vi "MeasureLeakageThreshold.vi"(5 "Junction Name":string, 6 "UiDefinition":T1, 7 ".NET Refnum":refnum<k24>, 8 "new file path (Not A Path if cancelled)":path, 9 "appended path":path, 11 ".NET Refnum in":refnum<k24>) -> (0 "error out":errorcluster)   [LabVIEW 2020]
uses:
  UIReferences.ctl
  C:/Users/User/Desktop/Automation/CurrentVersion/LabviewDXFViewer/bin/Release/LabviewDXFViewer.exe
  LabviewDXFViewer/bin/Release/LabviewDXFViewer.exe
  <vilib>/Utility/file.llb/Write Delimited Spreadsheet (string).vi
  <vilib>/Utility/file.llb/Write Delimited Spreadsheet (DBL).vi
panel:
  in  "CurrentPositionIndex":i32
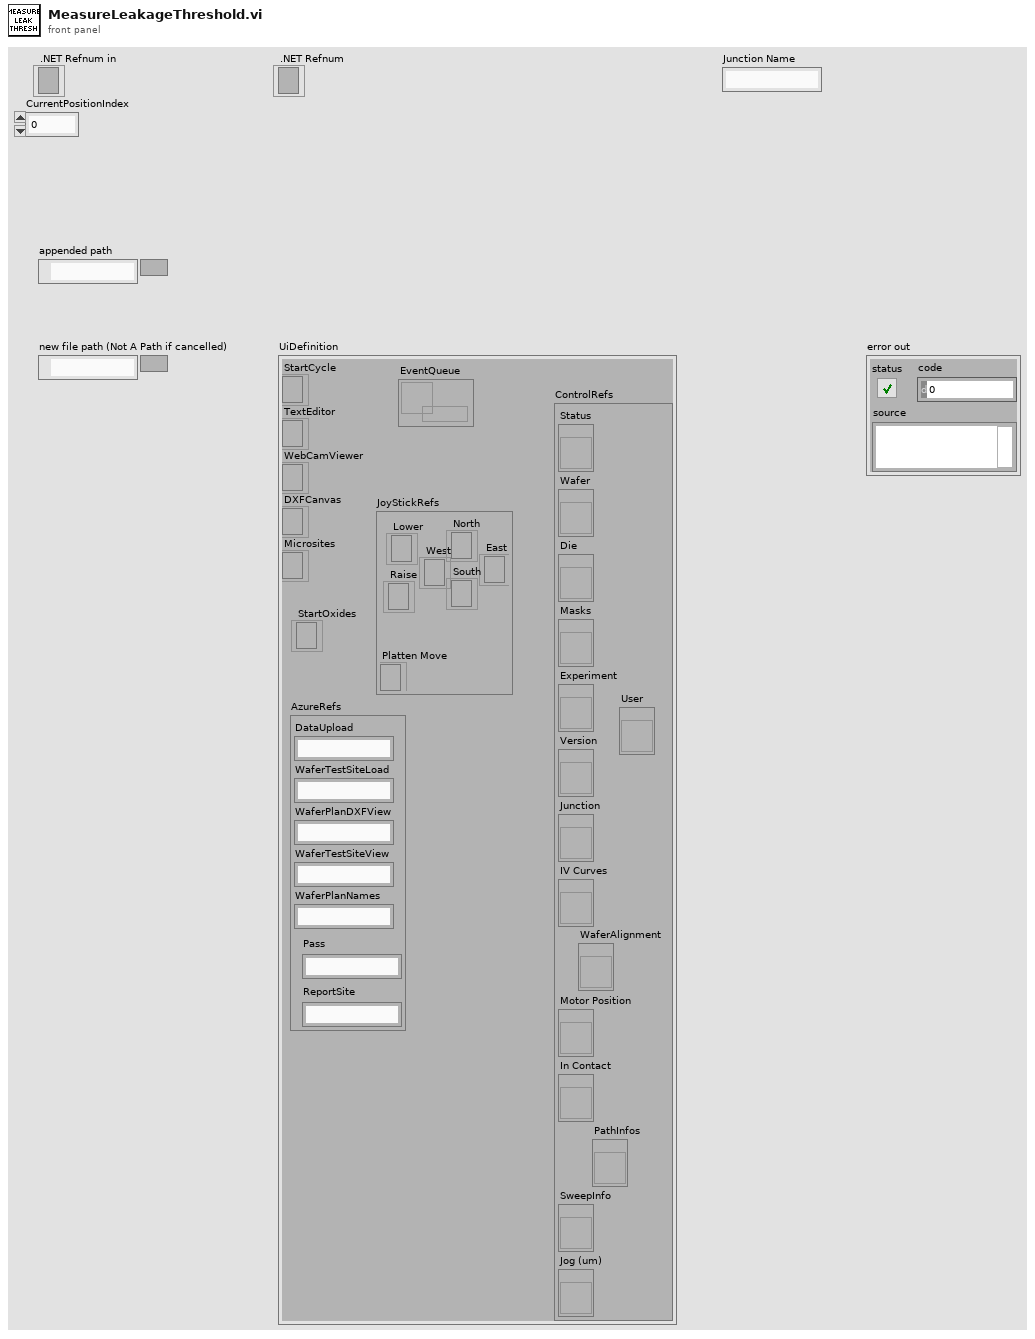
[diagram p1: front panel]
types:
  T1 = typedef "UIReferences.ctl" = cluster{"StartCycle":refnum<k24>, "TextEditor":refnum<k24>, "WebCamViewer":refnum<k24>, "DXFCanvas":refnum<k24>, "Microsites":refnum<k24>, "JoyStickRefs":cluster{"North":refnum<k24>, "Lower":refnum<k24>, "Raise":refnum<k24>, "Platten Move":refnum<k24>, "West":refnum<k24>, "East":refnum<k24>, "South":refnum<k24>}, "AzureRefs":cluster{"DataUpload":string, "WaferTestSiteLoad":string, "WaferPlanDXFView":string, "WaferTestSiteView":string, "WaferPlanNames":string, "Pass":string, "ReportSite":string}, "ControlRefs":cluster{"Status":refnum<vi>, "Wafer":refnum<vi>, "Die":refnum<vi>, "Masks":refnum<vi>, "Experiment":refnum<vi>, "Version":refnum<vi>, "Junction":refnum<vi>, "IV Curves":refnum<vi>, "Motor Position":refnum<vi>, "In Contact":refnum<vi>, "SweepInfo":refnum<vi>, "Jog (um)":refnum<vi>, "PathInfos":refnum<vi>, "User":refnum<vi>, "WaferAlignment":refnum<vi>}, "EventQueue":refnum<queue>, "StartOxides":refnum<k24>}
  T2 = typedef "CapacitanceInfos.ctl" = cluster{"Conductance":dbl, "CapacitanceIV":dbl, "Intercept":dbl, "CapacitanceSW":dbl, "Sum":dbl, "CapacitanceInfos":T3[], "CapacitancePhase":dbl, "dC/dV":dbl, "Function":string, "OtherInfo":dbl[][]}
  T3 = typedef "CapacitanceRecord.ctl" = cluster{"Freq":dbl, "Vpp":dbl, "PhaseS":dbl, "Irms":dbl, "PhaseC":dbl, "Theta":dbl, "VDrive":dbl, "Capacitance":dbl, "Other":dbl}
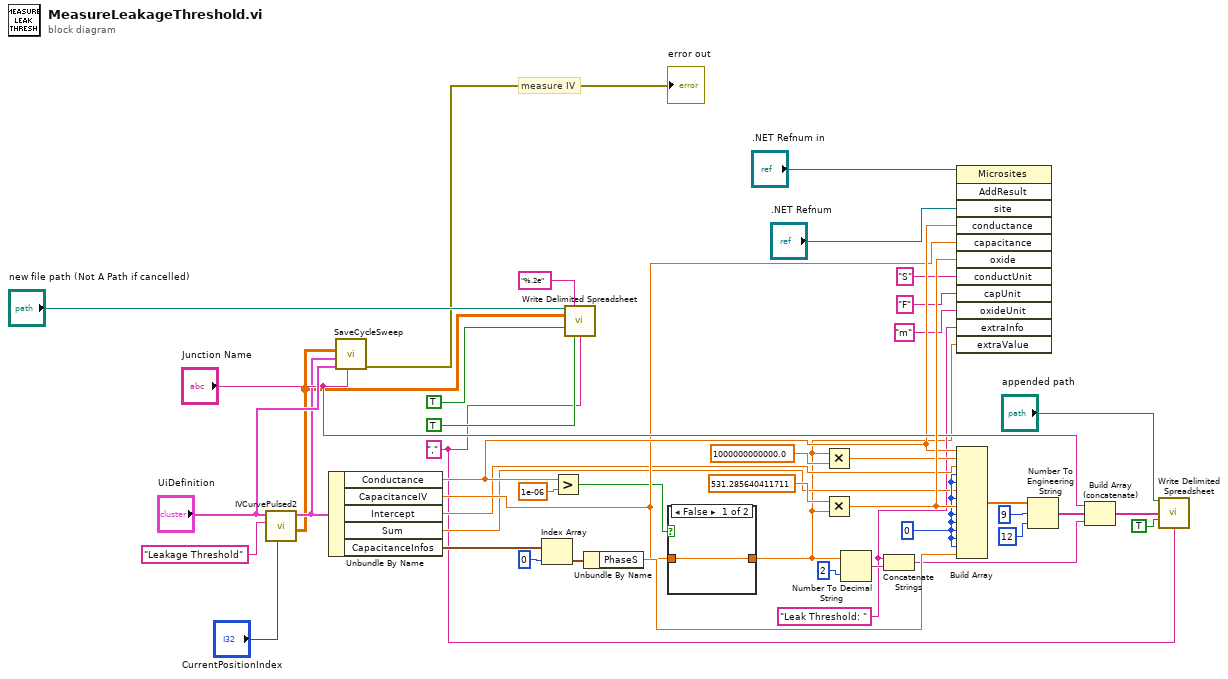
[diagram p0: block diagram]
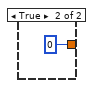
[diagram p2: hidden frame]
diagram:
  w3 = "Leak Threshold: "
  w8 = "," ("delimiter (\\t)")
  w41 = 0
  # "measure IV"
  n1 = call "IVCurvePulsed2.vi"("CurrentPositionIndex"="CurrentPositionIndex", "Program"="Leakage Threshold", "UiDefinition"="UiDefinition") -> ("appended array"=w16:dbl[][], "InfoCluster"=w29:T2)  [unwired: 7 in]
  n2 = Unbundle By Name(w29) -> ("Conductance"=w31:dbl, "CapacitanceIV"=w30:dbl, "Intercept"=w19:dbl, "Sum"=w20:dbl, "CapacitanceInfos"=w32:T3[])
  n3 = call "SaveCycleSweep.vi"("JunctionName"="Junction Name", "UiDefinition 2"="UiDefinition", "InfoCluster"=w29, "appended array"=w16) -> ("error out"=→"error out":errorcluster)  [unwired: 7 in]
  n4 = Index Array(array=w32, index=0) -> (element=w34:T3)
  n5 = Greater?(x=w31, y=1e-06) -> (0:w23:bool)
  n6 = call-poly <vilib>:"Write Delimited Spreadsheet.vi"("file path (dialog if empty)"="new file path (Not A Path if cancelled)", "format (%.3f)"="%.2e", "2D data"=w16, "append to file? (new file:F)"=TRUE, "transpose? (no:F)"=TRUE, "delimiter (\\t)"=w8) -> ()  [unwired: 8 in, 2 out]
  n7 = Unbundle By Name(w34) -> ("PhaseS"=w42:dbl)
  n8 = case shown="False" w23 {
    tunnel: [w45 0] -> w2
    tunnel: w30 -> [w45 _]
    frame False {
    }
    frame True {
    }
  }
  n9 = Multiply(x=w2, y=1000000000000.0) -> (x*y=w21:dbl)
  n10 = Multiply(x=531.285640411711, y=w2) -> (x*y=w44:dbl)
  n11 = Number To Decimal String(number=w2, width (-)=i16 2) -> (decimal integer string=w6:string)
  n12 = Concatenate Strings(w3, w6) -> (w4:string)
  n13 = invoke class="Microsites" method="AddResult"(reference=".NET Refnum in", "site"=".NET Refnum", "conductance"=w31, "capacitance"=w30, "oxide"=w44, "conductUnit"="S", "capUnit"="F", "oxideUnit"="m" ("interceptUnit"), "extraInfo"=w3, "extraValue"=w2) -> ()  [unwired: 2 in, 12 out]
  n14 = Build Array(w31, w21, w19, w41, w41, w20, w41, w44, w41, w41, w41, w41, w41, w42) -> (w18:dbl[])
  n15 = Number To Engineering String(2:i16 12 ("precision (6)"), 3:i16 9 ("width (-)"), 4:w18) -> (0:w10:string[])  [unwired: 1 in]
  n16 = Build Array (concatenate)("Junction Name", w10, w4) -> (w12:string[])
  n17 = call-poly <vilib>:"Write Delimited Spreadsheet.vi"("file path (dialog if empty)"="appended path", "1D data"=w12, "append to file? (new file:F)"=TRUE, "delimiter (\\t)"=w8) -> ()  [unwired: 10 in, 2 out]
